vi "AER2text.vi"() -> ()   [LabVIEW 2016]
uses:
  Cerebellum/Cerebellum.lvclass
  AER/AER.lvclass
panel:
  out "appended path":path
  in  "Right Hem Path":path=path "C:/Users/drPinzon/Downloads/biCNNprediction/Results/Grid/grid_3138213171/aer_00000.xml"
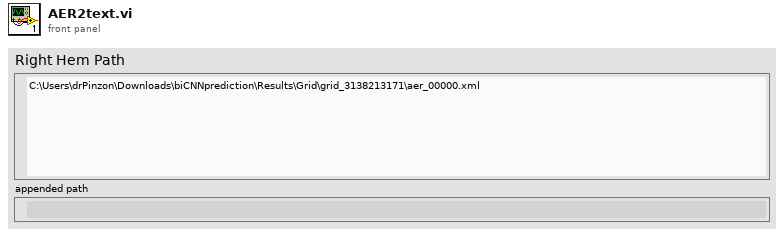
[diagram p1: front panel]
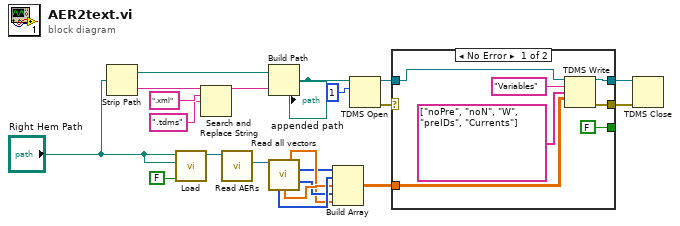
[diagram p0: block diagram]
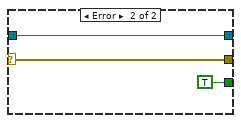
[diagram p2: hidden frame]
diagram:
  n1 = Strip Path(path="Right Hem Path") -> (stripped path=w17:path, name=w14:string)
  n2 = call "Load.vi"("Trained?"=FALSE, "Left Hem Path"="Right Hem Path", "Right Hem Path"="Right Hem Path") -> ("Cerebellum out"=w21:refnum<class "Cerebellum.lvclass">)  [unwired: 8 in]
  n3 = Search and Replace String(input string=w14, search string=".xml", replace string=".tdms" ("replace string (\"\")")) -> (result string=w15:string)  [unwired: 5 in, 3 out]
  n4 = call-dynamic "Read AERs.vi"("Cerebellum in"=w21) -> ("AER Left"=w10:refnum<class "AER.lvclass">)  [unwired: 7 in, 3 out]
  n5 = Build Path(base path=w17, name or relative path=w15) -> (appended path=w16:path)
  "appended path" <- w16
  n6 = call-dynamic "Read all vectors.vi"("AER in"=w10) -> ("Currents"=w6:dbl[], "No Pre"=w5:i32[], "Pre IDs"=w7:i32[], "No N"=w9:i32[], "W"=w8:dbl[])  [unwired: 4 in, 6 out]
  n7 = Build Array(w5, w9, w8, w7, w6) -> (w4:dbl[][])
  n8 = TDMS Open(10:i16 1 ("width (-)"), 11:w16) -> (0:w11:errorcluster, 3:w1:refnum<k34>)  [unwired: 5 in]
  n9 = case shown="No Error" w11 {
    selector: w11 -> [_ w29]
    tunnel: [w28 w30] -> w2
    tunnel: [w27 w29] -> w3
    tunnel: [FALSE TRUE] -> _
    tunnel: w4 -> [w23 _]
    tunnel: w1 -> [w22 w30]
    frame No Error {
      n10 = TDMS Write(0:w22, 5:"Variables" ("group name in (Untitled)"), 7:string[] ["noPre", "noN", "W", "preIDs", "Currents"] ("channel name(s) in (Untitled)"), 9:w23) -> (4:w28:refnum<k34>, 15:w27:errorcluster)  [unwired: 2 in, 2 out]
    }
    frame Error {
    }
  }
  n11 = TDMS Close(8:w3, 11:w2) -> ()  [unwired: 2 out]
